vi "R_core.vi"(1 "install path":path=path "C:/Program Files (x86)/National Instruments/LabLinda", 2 "OP":T1, 5 "IN VARIANT":variant, 7 "Ip":string, 9 "Name in":string, 11 "error in (no error)":errorcluster) -> (6 "OUT VARIANT":variant, 10 "Operation Ok":bool, 15 "error out":errorcluster)   [LabVIEW 2015]
doc: "REMOTE OUT"
uses:
  LI_states.ctl
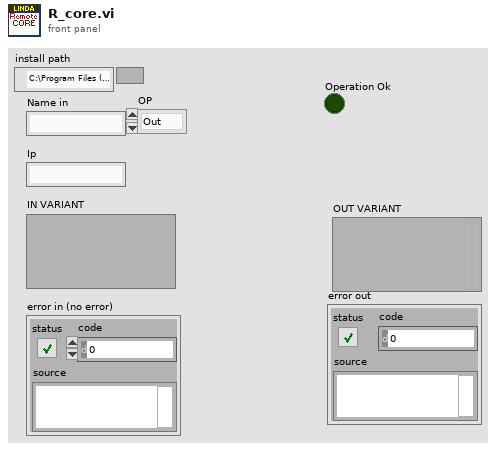
[diagram p1: front panel]
types:
  T1 = typedef "LI_states.ctl" = enum16{"Out", "In", "Rd", "Inp", "Rdp", "Init", "Cleanup", "RdAll"}
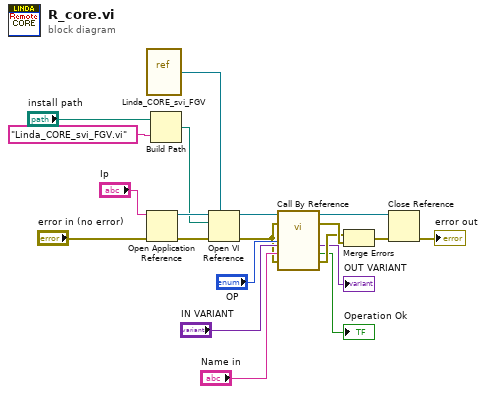
[diagram p0: block diagram]
diagram:
  n1 = vi-ref "Linda_CORE_svi_FGV.vi"() -> (w11:refnum<vi>)
  n2 = Open Application Reference(8:"error in (no error)", 11:"Ip") -> (0:w15:errorcluster, 3:w18:refnum<vi>)  [unwired: 2 in]
  n3 = Build Path(base path="install path", name or relative path="Linda_CORE_svi_FGV.vi") -> (appended path=w16:path)
  n4 = Open VI Reference(type specifier VI Refnum (for type only)=w11, application reference (local)=w18, vi path=w16, error in (no error)=w15) -> (vi reference=w10:refnum<vi>, error out=w6:errorcluster)  [unwired: 2 in]
  n5 = call-by-ref "?"(reference=w10, error in=w6, "OP"="OP", 8:"error in (no error)"=w6, "Name in"="Name in", "IN VARIANT"="IN VARIANT") -> (reference out=w3:refnum<vi>, error out=w5:errorcluster, 0:"error out"=w4:errorcluster, "Valid Op"=→"Operation Ok":bool, "OUT VARIANT"=→"OUT VARIANT":variant)  [unwired: 4 in, 1 out]
  n6 = Merge Errors(w4, w5) -> (w14:errorcluster)
  n7 = Close Reference(reference=w3, error in (no error)=w14) -> (error out=→"error out":errorcluster)
